vi "VerifConfigState.vi"(8 "error in (no error)":errorcluster, 11 "S4GUI in":refnum<class "S4GUI.lvclass">) -> (0 "error out":errorcluster, 3 "S4GUI out":refnum<class "S4GUI.lvclass">)   [LabVIEW 2018, in "S4GUI.lvclass"]
uses:
  S4GUI/S4GUI.lvclass
  S4GUI/S4GUI.lvclass/S4GUI.ctl
  Acquisition/Acquisition.lvclass
  Instrument/Instrument.lvclass
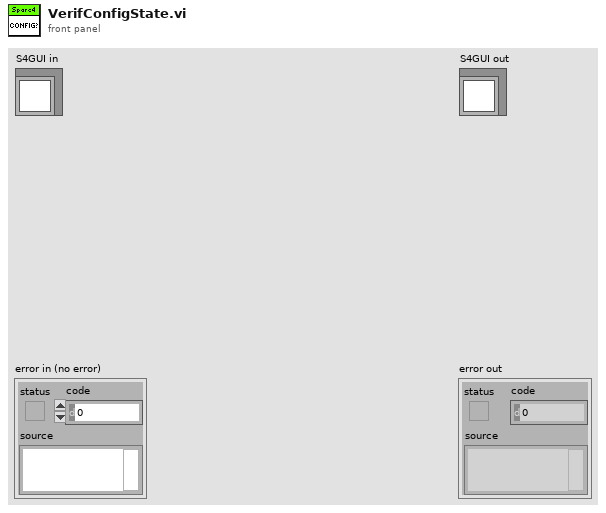
[diagram p1: front panel]
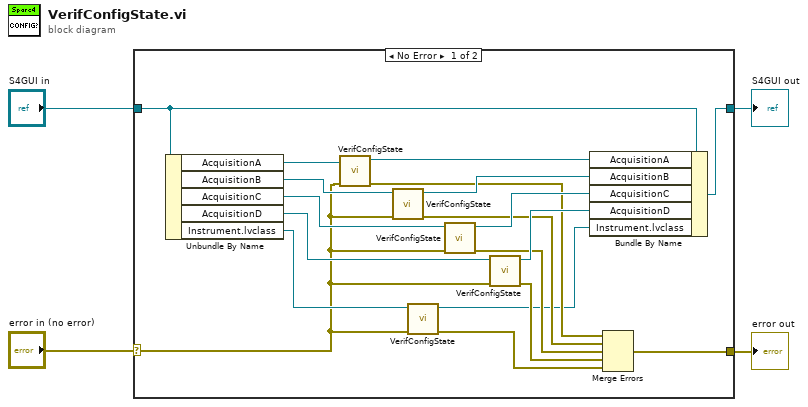
[diagram p0: block diagram]
diagram:
  n1 = case shown="No Error" "error in (no error)" {
    selector: "error in (no error)" -> [w5 w25]
    tunnel: [w9 w25] -> w3
    tunnel: [w18 w24] -> w1
    tunnel: "S4GUI in" -> [w19 w24]
    frame No Error {
      n2 = Unbundle By Name(w19) -> ("AcquisitionA"=w23:refnum<class "Acquisition.lvclass">, "AcquisitionB"=w22:refnum<class "Acquisition.lvclass">, "AcquisitionC"=w21:refnum<class "Acquisition.lvclass">, "AcquisitionD"=w20:refnum<class "Acquisition.lvclass">, "Instrument.lvclass"=w8:refnum<class "Instrument.lvclass">)
      n3 = call-dynamic "VerifConfigState.vi"("error in (no error)"=w5, "Acquisition in"=w23) -> ("error out"=w13:errorcluster, "Acquisition out"=w17:refnum<class "Acquisition.lvclass">)  [unwired: 8 in]
      n4 = call-dynamic "VerifConfigState.vi"("error in (no error)"=w5, "Acquisition in"=w22) -> ("error out"=w12:errorcluster, "Acquisition out"=w16:refnum<class "Acquisition.lvclass">)  [unwired: 8 in]
      n5 = call-dynamic "VerifConfigState.vi"("error in (no error)"=w5, "Instrument in"=w8) -> ("error out"=w6:errorcluster, "Instrument out"=w7:refnum<class "Instrument.lvclass">)  [unwired: 8 in]
      n6 = call-dynamic "VerifConfigState.vi"("error in (no error)"=w5, "Acquisition in"=w21) -> ("error out"=w11:errorcluster, "Acquisition out"=w15:refnum<class "Acquisition.lvclass">)  [unwired: 8 in]
      n7 = call-dynamic "VerifConfigState.vi"("error in (no error)"=w5, "Acquisition in"=w20) -> ("error out"=w10:errorcluster, "Acquisition out"=w14:refnum<class "Acquisition.lvclass">)  [unwired: 8 in]
      n8 = Bundle By Name(cluster=w19, "AcquisitionA"=w17, "AcquisitionB"=w16, "AcquisitionC"=w15, "AcquisitionD"=w14, "Instrument.lvclass"=w7) -> (w18:refnum<class "S4GUI.lvclass">)
      n9 = Merge Errors(w13, w12, w11, w10, w6) -> (w9:errorcluster)
    }
    frame Error {
    }
  }
  "error out" <- w3
  "S4GUI out" <- w1
